vi "baseline_scanV2.vi"() -> ()   [LabVIEW 2017] (continued)
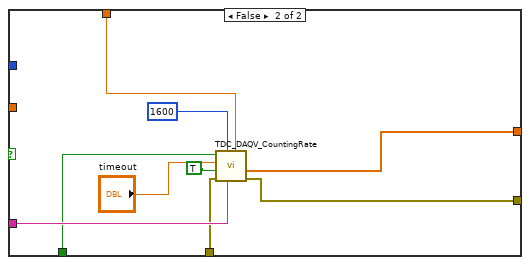
[diagram p3: hidden frame]
          n16 = call "TDC_DAQV_CountingRate.vi"("Thresholds (mV)"=w66, "address"=w70, "bytes to read"=1600, "error in (no error)"=w64, "UDP Config"=FALSE ("one key for threshold"), "SMA mode"=w63) -> ("error out"=w69:errorcluster, "rate_array"=w55:dbl[])  [unwired: 2 in, 2 out]
          n17 = Multiply(x=2, y=w60) -> (x*y=w56:i32)
          n18 = Index Array(array=w55, index=w56) -> (element=w61:dbl)
          n19 = Increment(x=w56) -> (x+1=w53:i32)
          n20 = Replace Array Subset(array=w62, new element=w61, index=w56) -> (w58:dbl[])
          n21 = Index Array(array=w55, index=w53) -> (element=w54:dbl)
          n22 = Replace Array Subset(array=w58, new element=w54, index=w53) -> (w57:dbl[])
          "current channel" <- w60
        }
      }
      frame False {
        n23 = call "TDC_DAQV_CountingRate.vi"("Thresholds"=w76, "address"=w79, "bytes to read"=1600, "error in (no error)"=w73, "UDP Config"=TRUE ("one key for threshold"), "timeout"="timeout", "SMA mode"=w74) -> ("error out"=w78:errorcluster, "rate_array"=w77:dbl[])  [unwired: 1 in, 2 out]
      }
    }
    "error out" <- w37
    "cal" <- w28
    n24 = disable-structure shown="Disabled" {
      disable-tunnel: w40 -> [w93 _]
      disable-tunnel: w39 -> [w92 _]
      frame Disabled {
        n25 = property on="1000ps, 5 ns" class="XYGraph (strict)"("Active Plot"=w93, "Plot.Plot Name"=w92) -> ()  [unwired: 2 in, 2 out]
      }
      frame Enabled {
      }
    }
    n26 = for {
      tunnel: w28 -> [w89] mode=indexing
      shift-right: [w81] -> w34
      shift-left: w36 -> [w84]
      tunnel: w35 -> [w91]
      i -> [w83]
      n27 = Index Array(array=w84, index=w83) -> (element=w85:cluster{dbl[], dbl[]})
      n28 = Unbundle(w85) -> (w90:dbl[], w88:dbl[])
      n29 = Build Array (concatenate)(w90, w91) -> (w87:dbl[])
      n30 = Build Array (concatenate)(w88, w89) -> (w86:dbl[])
      n31 = Bundle(cluster=w85, w87, w86) -> (w82:cluster{dbl[], dbl[]})
      n32 = Replace Array Subset(array=w84, new element=w82, index=w83) -> (w81:cluster{dbl[], dbl[]}[])
    }
    "1000ps, 5 ns" <- w34
  }
  n33 = Initialize Array(-1.0 ("element"), 64 ("dimension size")) -> (w15:dbl[])
  n34 = for {
    tunnel: w8 -> [w107] mode=indexing
    shift-right: [w94] -> w12
    shift-left: w15 -> [w100]
    shift-right: [w95] -> w14
    shift-left: w15 -> [w96]
    tunnel: [w98] -> w13 mode=indexing
    i -> [w98]
    n35 = Unbundle(w107) -> (w105:dbl[], w106:dbl[])
    n36 = for {
      tunnel: w106 -> [w108] mode=indexing
      tunnel: w105 -> [w115]
      shift-right: [w113] -> w103
      shift-left: dbl[] [] -> [w114]
      i -> [w112]
      n37 = Not Equal?(x=w108, y=-1.0) -> (x != y?=w116:bool)
      n38 = Not Equal To 0?(x=w108) -> (x != 0?=w109:bool)
      n39 = And(x=w116, y=w109) -> (x .and. y?=w110:bool)
      n40 = case shown="True" w110 {
        tunnel: w115 -> [_ w122]
        tunnel: w114 -> [w117 w121]
        tunnel: [w117 w120] -> w113
        tunnel: w112 -> [_ w118]
        frame False {
        }
        frame True {
          n41 = Index Array(array=w122, index=w118) -> (element=w119:dbl)
          n42 = Build Array (concatenate)(w121, w119) -> (w120:dbl[])
        }
      }
    }
    n43 = Array Size(array=w103) -> (size(s)=w97:i32)
    n44 = Decrement(x=w97) -> (x-1=w102:i32)
    n45 = Index Array(array=w103) -> (element=w101:dbl)  [unwired: 1 in]
    n46 = Index Array(array=w103, index=w102) -> (element=w99:dbl)
    n47 = Replace Array Subset(array=w96, new element=w101, index=w98) -> (w95:dbl[])
    n48 = Replace Array Subset(array=w100, new element=w99, index=w98) -> (w94:dbl[])
  }
  n49 = Bundle(w13, w14) -> (w11:cluster{i32[], dbl[]})  [unwired: 1 in]
  n50 = Bundle(w13, w12) -> (w10:cluster{i32[], dbl[]})  [unwired: 1 in]
  n51 = Build Array(w11, w10) -> (→"result":cluster{i32[], dbl[]}[])
